vi "Test - Add  Property (String).vi"() -> ()   [LabVIEW 2020, in "JSON Schema Generator.lvlib"]
uses:
  <vilib>/JDP Science/JSONtext/LVClass Serializer/JSONtext LVClass Serializer.lvclass
  JSON Schema Generator.lvlib
  <vilib>/addons/_JKI Toolkits/Caraya/classes/Test/Test.lvclass
  <vilib>/addons/_JKI Toolkits/Caraya/classes/Assert/Assert.lvclass
  <vilib>/JDP Science/JSONtext/JSONtext.lvlib
  <vilib>/addons/_JKI Toolkits/Caraya/classes/Assert/Assert Equal Value_Variant.vi
  5e3b1551-949d-4aa0-a100-e726d27281b9.vi
  <vilib>/addons/_JKI Toolkits/Caraya/classes/Assert/Assert True.vi
  <vilib>/addons/_JKI Toolkits/Caraya/classes/Assert/Assert Not Error.vi
  50dbb99c-9102-4768-b381-ebef3ccadd32.vi
  75de3de8-465a-458e-8514-062b16a035d8.vi
  <vilib>/addons/_JKI Toolkits/Caraya/classes/Assert/Assert False.vi
panel:
  in  "String":string
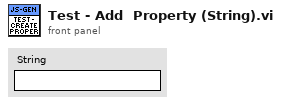
[diagram p1: front panel]
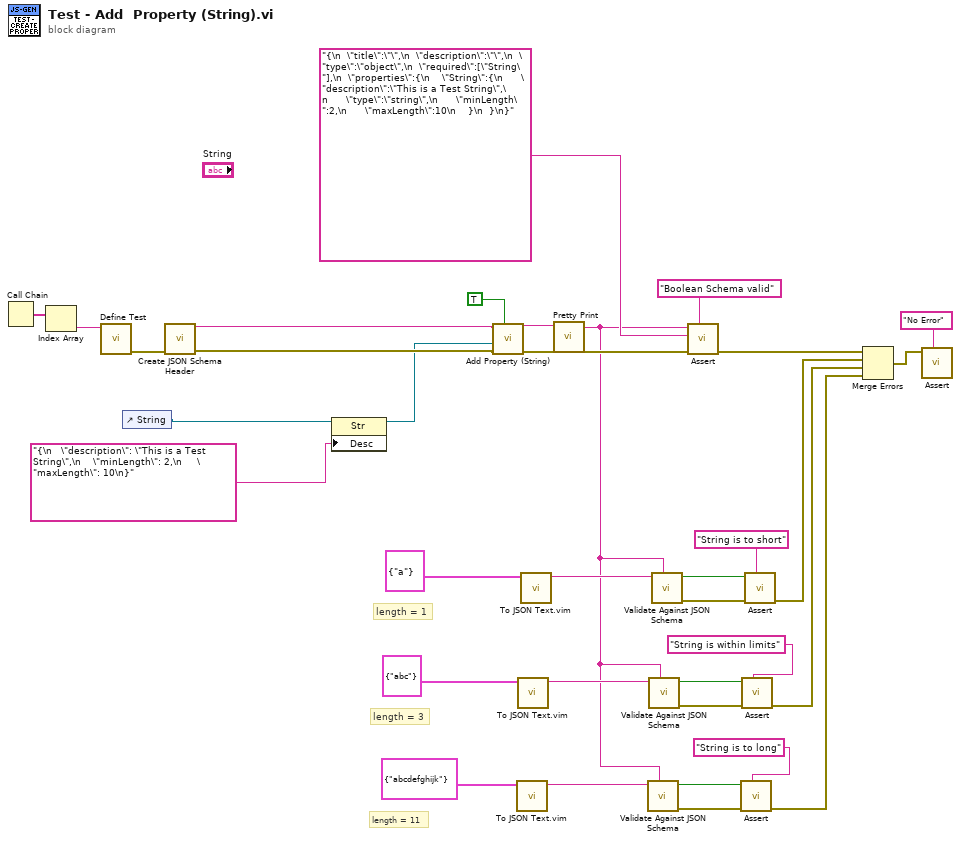
[diagram p0: block diagram]
diagram:
  # "length = 11"
  # "length = 3"
  # "length = 1"
  n1 = Call Chain() -> (call chain=w36:string[])
  n2 = Index Array(array=w36) -> (element=w35:string)  [unwired: 1 in]
  n3 = call <vilib>:"Define Test.vi"("Label (VI Title)"=w35) -> ("error out"=w31:errorcluster)  [unwired: 9 in, 1 out]
  n4 = control-ref of="String"() -> (w28:refnum<vi>)
  n5 = call "Create JSON Schema Header.vi"("error in (no error)"=w31) -> ("error out"=w26:errorcluster, "JSON Schema out"=w27:string)  [unwired: 9 in]
  n6 = property on="Property Node" class="Str"(reference=w28, "Desc"="{\n   \"description\": \"This is a Test String\",\n    \"minLength\": 2,\n     \"maxLength\": 10\n}" ("Description")) -> (reference out=w25:refnum<vi>)  [unwired: 1 in, 1 out]
  n7 = call "Add Property (String).vi"("Required?"=TRUE, "error in (no error)"=w26, "String In"=w25, "JSON Schema in"=w27) -> ("error out"=w22:errorcluster, "JSON SChema out"=w23:string)  [unwired: 6 in]
  n8 = call "To JSON Text.vim"("Anything"=cluster{"String":string} {"String"="abcdefghijk"}) -> ("<JSON>"=w8:string)  [unwired: 9 in, 1 out]
  n9 = call "To JSON Text.vim"("Anything"=cluster{"String":string} {"String"="abc"}) -> ("<JSON>"=w11:string)  [unwired: 9 in, 1 out]
  n10 = call "To JSON Text.vim"("Anything"=cluster{"String":string} {"String"="a"}) -> ("<JSON>"=w19:string)  [unwired: 9 in, 1 out]
  n11 = call <vilib>:"Pretty Print.vi"("error in (no error)"=w22, "JSON"=w23) -> ("error out"=w30:errorcluster, "<JSON>"=w3:string)  [unwired: 7 in, 1 out]
  n12 = call <vilib>:"Validate Against JSON Schema.vi"("JSON Schema"=w3, "JSON"=w8) -> ("error out"=w6:errorcluster, "Invalid"=w7:bool)  [unwired: 5 in, 3 out]
  n13 = call <vilib>:"Validate Against JSON Schema.vi"("JSON Schema"=w3, "JSON"=w11) -> ("error out"=w13:errorcluster, "Invalid"=w12:bool)  [unwired: 5 in, 3 out]
  n14 = call <vilib>:"Validate Against JSON Schema.vi"("JSON Schema"=w3, "JSON"=w19) -> ("error out"=w15:errorcluster, "Invalid"=w18:bool)  [unwired: 5 in, 3 out]
  n15 = call-poly <vilib>:"Assert.vi"("Label"="Boolean Schema valid", "error in (no error)"=w30, "Actual"="{\n  \"title\":\"\",\n  \"description\":\"\",\n  \"type\":\"object\",\n  \"required\":[\"String\"],\n  \"properties\":{\n    \"String\":{\n      \"description\":\"This is a Test String\",\n      \"type\":\"string\",\n      \"minLength\":2,\n      \"maxLength\":10\n    }\n  }\n}", "Expected"=w3) -> ("error out"=w33:errorcluster)  [unwired: 6 in, 1 out]
  n16 = call-poly <vilib>:"Assert.vi"("Label"="String is to long", "error in (no error)"=w6, "True?"=w7) -> ("error out"=w4:errorcluster)  [unwired: 7 in, 1 out]
  n17 = call-poly <vilib>:"Assert.vi"("Label"="String is within limits", "error in (no error)"=w13, "False?"=w12) -> ("error out"=w5:errorcluster)  [unwired: 7 in, 1 out]
  n18 = call-poly <vilib>:"Assert.vi"("Label"="String is to short", "error in (no error)"=w15, "True?"=w18) -> ("error out"=w16:errorcluster)  [unwired: 7 in, 1 out]
  n19 = Merge Errors(w33, w16, w5, w4) -> (w17:errorcluster)
  n20 = call-poly <vilib>:"Assert.vi"("Label"="No Error", "Not Error?"=w17) -> ()  [unwired: 8 in, 2 out]
